vi "PF_STRING_DATA (SubVI).vi"(9 "Value":bool[](array[boolean]), 10 "Value 2":dbl, 11 "Value 3":dbl) -> (3 "String":string)   [LabVIEW 2020]
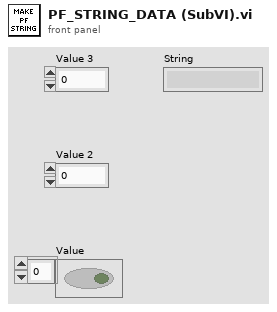
[diagram p1: front panel]
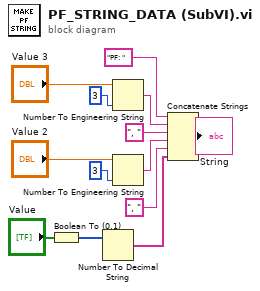
[diagram p0: block diagram]
diagram:
  n1 = Boolean To (0,1)(Boolean="Value") -> (0, 1=w11:i16[])
  n2 = Number To Decimal String(number=w11) -> (decimal integer string=w12:string[])  [unwired: 1 in]
  n3 = Number To Engineering String(2:i16 3 ("precision (6)"), 4:"Value 3") -> (0:w1:string)  [unwired: 2 in]
  n4 = Number To Engineering String(2:i16 3 ("precision (6)"), 4:"Value 2") -> (0:w3:string)  [unwired: 2 in]
  n5 = Concatenate Strings("PF: ", w1, ", ", w3, ", ", w12) -> (→"String":string)
